vi "LS 3XX setT.vi"(7 "instrument":enum16{"336", "340"}(ring), 8 "power":enum16{"no change", "off", "low", "med", "high"}(ring), 9 "setT":dbl=70.0, 10 "loop":enum16{"1", "2"}(ring)=enum."2", 11 "GPIB":refnum<visa-resource-name>="GPIB0::12::INSTR") -> ()   [LabVIEW 2025]
panel:
  out "concatenated string":string
  out "error out":errorcluster
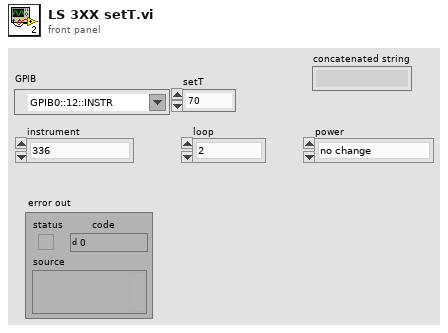
[diagram p1: front panel]
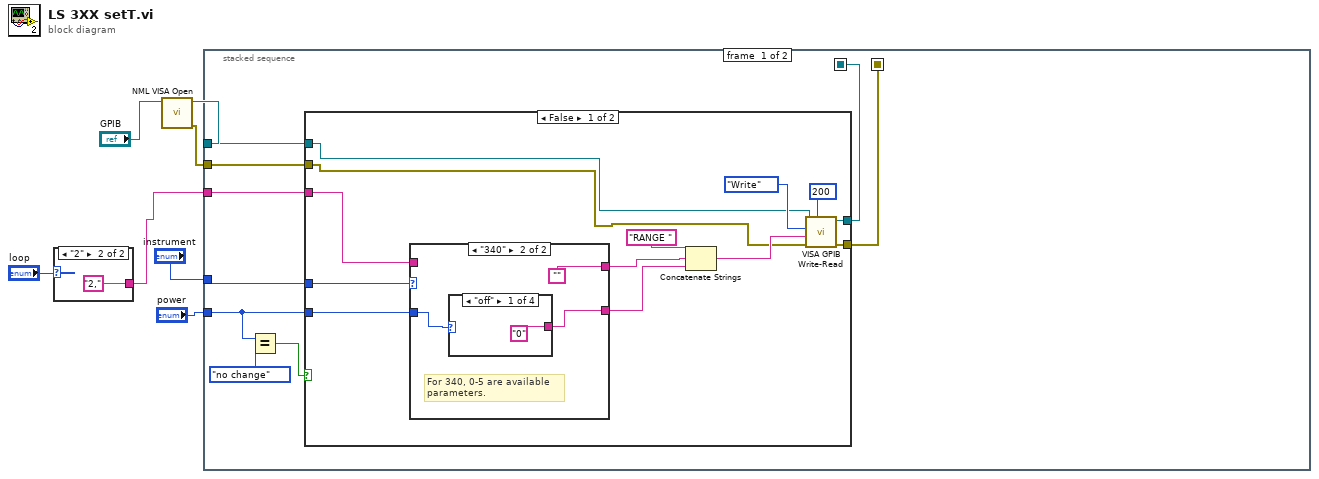
[diagram p0: block diagram]
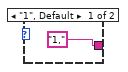
[diagram p2: hidden frame]
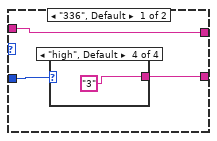
[diagram p3: hidden frame]
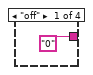
[diagram p4: hidden frame]
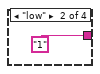
[diagram p5: hidden frame]
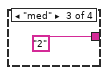
[diagram p6: hidden frame]
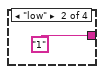
[diagram p7: hidden frame]
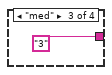
[diagram p8: hidden frame]
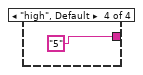
[diagram p9: hidden frame]
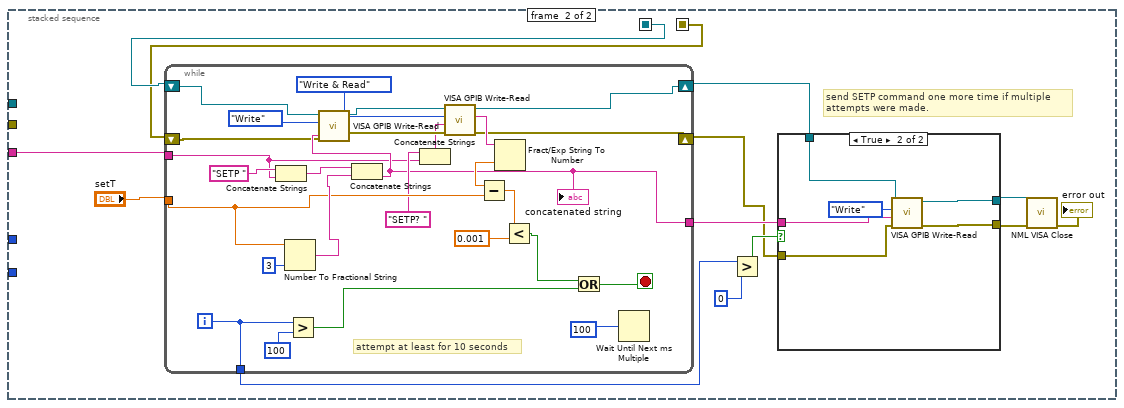
[diagram p11: hidden frame]
diagram:
  n1 = case shown="\"2\"" "loop" {
    tunnel: ["1," ("loop") "2," ("loop")] -> w4
    frame "1", Default {
    }
    frame "2" {
    }
  }
  n2 = call "NML VISA Open.vi"("VISA resource name"="GPIB") -> ("error out"=w2:errorcluster, "VISA resource name out"=w6:refnum<visa-resource-name>)  [unwired: 9 in]
  n3 = stacked-sequence {
    seq-local: [w17 _] -> [_ w53]
    seq-local: [w15 _] -> [_ w49]
    tunnel: w6 -> [w18 _]
    tunnel: w4 -> [w16 w59]
    tunnel: "instrument" -> [w13 _]
    tunnel: w2 -> [w14 _]
    tunnel: "power" -> [w12 _]
    frame #0 {
      n4 = Equal?(x=w12, y=enum16{"no change", "off", "low", "med", "high"}."no change") -> (x = y?=w10:bool)
      n5 = case shown="False" w10 {
        tunnel: w18 -> [w27 w47]
        tunnel: [w26 w47] -> w17
        tunnel: w13 -> [w24 _]
        tunnel: w16 -> [w22 _]
        tunnel: [w21 w46] -> w15
        tunnel: w14 -> [w20 w46]
        tunnel: w12 -> [w19 _]
        frame False {
          n6 = case shown="\"340\"" w24 {
            tunnel: [w34 w39] -> w29
            tunnel: w19 -> [w33 w40]
            tunnel: [w32 ""] -> w23
            tunnel: w22 -> [w32 _]
            frame "336", Default {
              n7 = case shown="\"high\", Default" w33 {
                tunnel: ["0" ("format string") "1" ("format string") "2" ("format string") "3" ("format string")] -> w34
                frame "off" {
                }
                frame "low" {
                }
                frame "med" {
                }
                frame "high", Default {
                }
              }
            }
            frame "340" {
              # "For 340, 0-5 are available\nparameters."
              n8 = case shown="\"off\"" w40 {
                tunnel: ["0" ("format string") "1" ("format string") "3" ("format string") "5" ("format string")] -> w39
                frame "off" {
                }
                frame "low" {
                }
                frame "med" {
                }
                frame "high", Default {
                }
              }
            }
          }
          n9 = Concatenate Strings("RANGE " ("format string"), w23, w29) -> (w28:string)
          n10 = call "VISA GPIB Write-Read.vi"("Wait (ms)"=u32 200 ("wait (mS)"), "error in (no error)"=w20, "Command"=w28, "Action"=enum16{"Write", "Read", "Write & Read"}."Write", "VISA resource name"=w27) -> ("error out"=w21:errorcluster, "dup VISA Session"=w26:refnum<visa-resource-name>)  [unwired: 3 in, 2 out]
        }
        frame True {
        }
      }
    }
    frame #1 {
      # "send SETP command one more time if multiple\nattempts were made."
      n11 = while {
        tunnel: "setT" -> [w87]
        tunnel: w59 -> [w69]
        tunnel: [w77] -> w58
        tunnel: [w75] -> w55
        shift-right: [w73] -> w54
        shift-left: w49 -> [w74]
        shift-right: [w71] -> w52
        shift-left: w53 -> [w72]
        i -> [w77]
        stop <- w80 stop-if-true
        # "attempt at least for 10 seconds"
        n12 = Concatenate Strings("SETP " ("Command"), w69) -> (w85:string)
        n13 = Number To Fractional String(number=w87, precision (6)=i16 3) -> (F-format string=w94:string)  [unwired: 2 in]
        n14 = Greater?(x=w77, y=100) -> (0:w81:bool)
        n15 = Concatenate Strings(w85, w94) -> (w75:string)
        "concatenated string" <- w75
        n16 = call "VISA GPIB Write-Read.vi"("error in (no error)"=w74, "Command"=w75, "Action"=enum16{"Write", "Read", "Write & Read"}."Write", "VISA resource name"=w72) -> ("error out"=w79:errorcluster, "dup VISA Session"=w93:refnum<visa-resource-name>)  [unwired: 4 in, 2 out]
        n17 = Concatenate Strings("SETP? " ("Command"), w69) -> (w76:string)
        n18 = call "VISA GPIB Write-Read.vi"("error in (no error)"=w79, "Command"=w76, "Action"=enum16{"Write", "Read", "Write & Read"}."Write & Read", "VISA resource name"=w93) -> ("error out"=w73:errorcluster, "String Returned"=w91:string, "dup VISA Session"=w71:refnum<visa-resource-name>)  [unwired: 4 in, 1 out]
        n19 = Fract/Exp String To Number(string=w91) -> (number=w90:dbl)  [unwired: 3 in, 1 out]
        n20 = Subtract(x=w90, y=w87) -> (x-y=w89:dbl)
        n21 = Less?(x=w89, y=0.001) -> (x < y?=w82:bool)
        n22 = Or(x=w82, y=w81) -> (x .or. y?=w80:bool)
        n23 = Wait Until Next ms Multiple(millisecond multiple=u32 100) -> ()  [unwired: 1 out]
      }
      n24 = Greater?(x=w58, y=0) -> (0:w56:bool)
      n25 = case shown="True" w56 {
        tunnel: w52 -> [w61 w68]
        tunnel: w55 -> [_ w66]
        tunnel: w54 -> [w62 w65]
        tunnel: [w62 w64] -> w50
        tunnel: [w61 w63] -> w51
        frame False {
        }
        frame True {
          n26 = call "VISA GPIB Write-Read.vi"("error in (no error)"=w65, "Command"=w66, "Action"=enum16{"Write", "Read", "Write & Read"}."Write", "VISA resource name"=w68) -> ("error out"=w64:errorcluster, "dup VISA Session"=w63:refnum<visa-resource-name>)  [unwired: 4 in, 2 out]
        }
      }
      n27 = call "NML VISA Close.vi"("Error In"=w50, "VISA resource name"=w51) -> ("Error Out"=→"error out":errorcluster)  [unwired: 9 in]
    }
  }
